vi "DCS_write_signal_hdf5.vi"(7 "Index":u64, 8 "error in":errorcluster, 10 "Save Path":path, 11 "Signal array":T2(array[cluster])) -> (0 "error out":errorcluster)   [LabVIEW 2013]
uses:
  User Interface/Controls/Role ID.ctl
  <vilib>/addons/h5labview/polymorph/H5D_write_var.vi
  <vilib>/addons/h5labview/H5Dataset.lvlib
  <vilib>/addons/h5labview/H5Attrib.lvlib
  <vilib>/addons/h5labview/H5File.lvlib
panel:
  out "concatenated string":string
  out "Role ID":T1
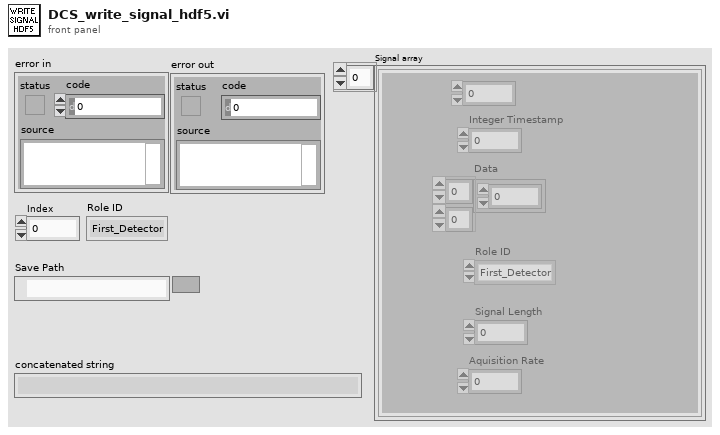
[diagram p1: front panel]
types:
  T1 = typedef "Role ID.ctl" = enum16{"First_Detector", "Second_Detector", "Third_Detector", "LeCroy_CH1", "LeCroy_CH2", "LeCroy_CH3", "LeCroy_CH4", "PSU", "DCS 1", "DCS 2"}
  T2 = cluster{"Data":dbl[][], "Integer Timestamp":u64, "Signal Length":u32, "DCS_ID":u32, "Role ID":T1, "Aquisition Rate":dbl}[]
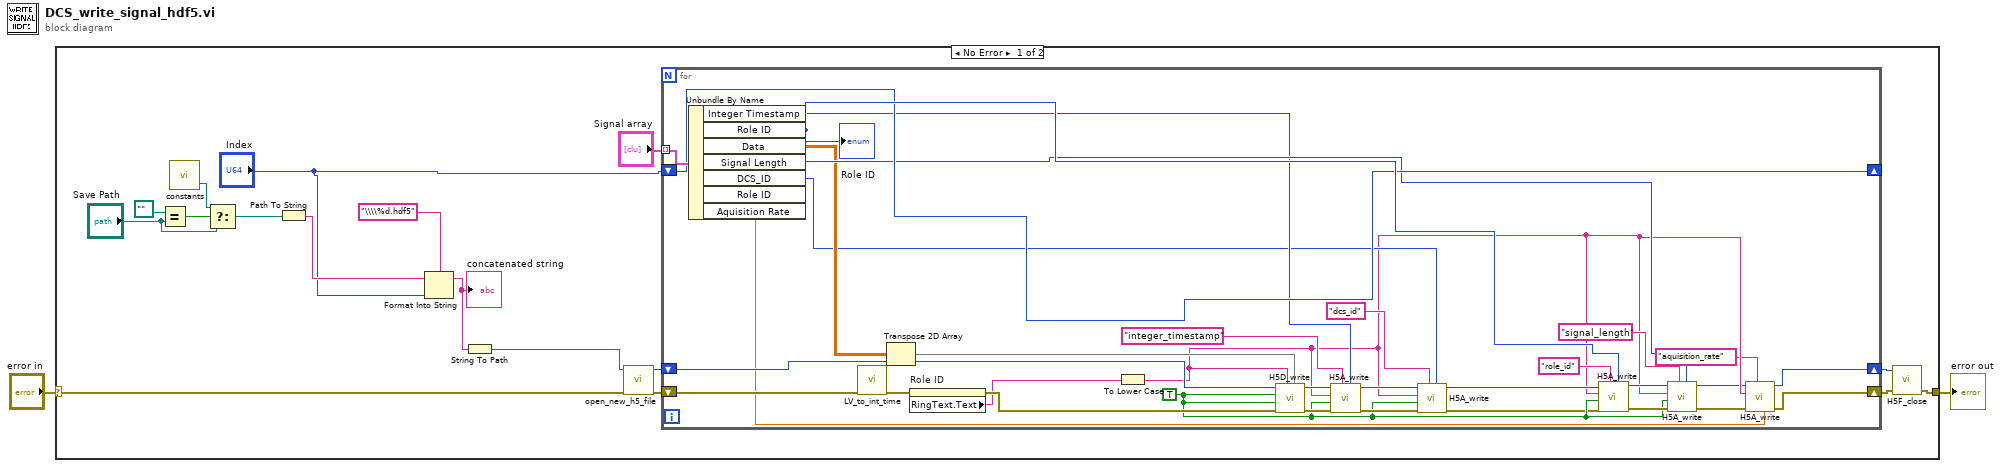
[diagram p0: block diagram]
diagram:
  n1 = case shown="No Error" "error in" {
    selector: "error in" -> [w3 w53]
    tunnel: [w14 w53] -> w1
    frame No Error {
      n2 = Equal?(x=path "" ("Save Path"), y="Save Path") -> (x = y?=w11:bool)
      n3 = call "constants.vi"() -> ("Processed HDF5 filepath"=w8:path)  [unwired: 3 out]
      n4 = Select(t=w8, s=w11, f="Save Path") -> (s? t:f=w13:path)
      n5 = Path To String(path=w13) -> (string=w5:string)
      n6 = Format Into String(format string="\\\\%d.hdf5", initial string=w5, "Index") -> (resulting string=w6:string)  [unwired: 1 in, 1 out]
      "concatenated string" <- w6
      n7 = String To Path(string=w6) -> (path=w9:path)
      n8 = call "open_new_h5_file.vi"("error in (no error)"=w3, "path"=w9) -> ("error out"=w18:errorcluster, "ref"=w17:i32)  [unwired: 8 in]
      n9 = for {
        tunnel: "Signal array" -> [w52] mode=indexing
        shift-right: [w25] -> w15
        shift-left: w18 -> [w51]
        shift-right: [w34] -> _
        shift-left: "Index" -> [w34]
        shift-right: [w21] -> w16
        shift-left: w17 -> [w49]
        w36 = TRUE ("preserve attribs?")
        n10 = Unbundle By Name(w52) -> ("Integer Timestamp"=w30:u64, "Role ID"=w41:T1, "Data"=w29:dbl[][], "Signal Length"=w31:u32, "DCS_ID"=w27:u32, "Aquisition Rate"=w20:dbl)  [unwired: 1 out]
        "Role ID" <- w41
        n11 = call "LV_to_int_time.vi"("error in (no error)"=w51) -> ("error out"=w50:errorcluster)  [unwired: 8 in, 1 out]
        n12 = Transpose 2D Array(2D array=w29) -> (transposed array=w28:dbl[][])
        n13 = property on="Role ID" class="Enum (strict)"(error in=w50) -> (error out=w48:errorcluster, "RingText.Text"=w35:string)  [unwired: 1 in, 1 out]
        n14 = To Lower Case(string=w35) -> (all lower case string=w24:string)
        n15 = call-poly <vilib>:"H5D_write.vi"("data"=w28, "name"=w24, "error in (no error)"=w48, "overwrite?"=w36, "preserve attribs?"=w36, "ref"=w49) -> ("error out"=w46:errorcluster, "ref out"=w47:i32)  [unwired: 2 in]
        n16 = call <vilib>:"H5A_write.vi"("value"=w30, "attrib_name"="integer_timestamp", "error in (no error)"=w46, "overwrite? (F)"=w36, "obj_name"=w24, "ref"=w47) -> ("error out"=w39:errorcluster, "ref out"=w38:i32)  [unwired: 2 in]
        n17 = call <vilib>:"H5A_write.vi"("value"=w27, "attrib_name"="dcs_id", "error in (no error)"=w39, "overwrite? (F)"=w36, "obj_name"=w24, "ref"=w38) -> ("error out"=w33:errorcluster, "ref out"=w32:i32)  [unwired: 2 in]
        n18 = call <vilib>:"H5A_write.vi"("value"=w41, "attrib_name"="role_id", "error in (no error)"=w33, "overwrite? (F)"=w36, "obj_name"=w24, "ref"=w32) -> ("error out"=w40:errorcluster, "ref out"=w37:i32)  [unwired: 2 in]
        n19 = call <vilib>:"H5A_write.vi"("value"=w31, "attrib_name"="signal_length", "error in (no error)"=w40, "overwrite? (F)"=w36, "obj_name"=w24, "ref"=w37) -> ("error out"=w26:errorcluster, "ref out"=w22:i32)  [unwired: 2 in]
        n20 = call <vilib>:"H5A_write.vi"("value"=w20, "attrib_name"="aquisition_rate", "error in (no error)"=w26, "obj_name"=w24, "ref"=w22) -> ("error out"=w25:errorcluster, "ref out"=w21:i32)  [unwired: 3 in]
      }
      n21 = call <vilib>:"H5F_close.vi"("error in (no error)"=w15, "ref"=w16) -> ("error out"=w14:errorcluster)  [unwired: 3 in]
    }
    frame Error {
    }
  }
  "error out" <- w1
